vi "Counter - Read Pulse Duty Cycle and Frequency (Continuous).vi"() -> ()   [LabVIEW 2022 SP3]
doc: "This example demonstrates how to configure a Pulse measurement to acquire frequency and duty cycle based off of an external clock. \n\nThe pulse measurement feature was introduced with NI X Series and 2nd generation NI CompactDAQ devices.\n\nFor instructions on how to connect your signals to the DAQ device, refer to your device documentation."
uses:
  <vilib>/Utility/error.llb/DialogType.ctl
  <vilib>/DAQmx/read.llb/DAQmx Read (Counter 1D Pulse Freq 1 Chan NSamp).vi
  <vilib>/DAQmx/create/channels.llb/DAQmx Create Channel (CI-Pulse Freq).vi
  <vilib>/DAQmx/configure/timing.llb/DAQmx Timing (Sample Clock).vi
  <vilib>/DAQmx/miscellaneous.llb/DAQmx Fill In Error Info.vi
  <resource>/objmgr/daqmx.rc
panel:
  out "Data Array":cluster{"Duty Cycle":dbl, "Frequency":dbl}[](array[cluster])
  in  "Sample Rate":dbl=1000.0
  in  "External Clock Source":tag="PFI0"
  in  "Min Frequency":dbl=2.0 format="%0.6f"
  in  "Max Frequency":dbl=100.0 format="%0.6f"
  in  "Pulse Frequency Terminal":tag="PFI9"
  in  "Stop":bool
  in  "Samples per Loop":i32=1000
  in  "Counter":tag="Dev1/ctr0"
  # "Channel Settings"
  # "Acquired Data"
  # "Timing Settings"
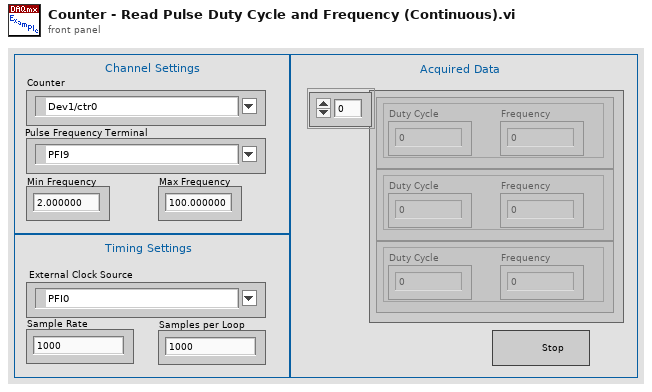
[diagram p1: front panel]
types:
  T1 = typedef "DialogType.ctl" = u16
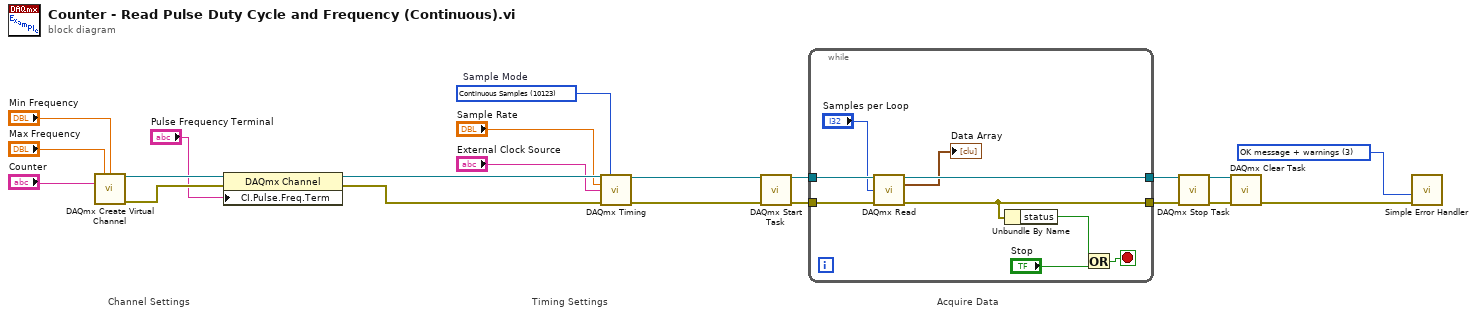
[diagram p0: block diagram]
diagram:
  w1 = T1 3 items=["no dialog", "OK message", "continue or stop message", "OK message + warnings", "continue/stop + warnings"] ("type of dialog (OK msg:1)")
  w21 = 10123 items=["Finite Samples"=10178, "Continuous Samples"=10123, "Hardware Timed Single Point"=12522]  # Sample Mode
  # "Acquire Data"
  # "Timing Settings"
  # "Channel Settings"
  n1 = call-poly <vilib>:"DAQmx Create Virtual Channel.vi"("maximum value"="Max Frequency", "minimum value"="Min Frequency", "counter"="Counter") -> ("task out"=w12:refnum<k21>, "error out"=w11:errorcluster)  [unwired: 11 in]
  n2 = property class="DAQmx Channel"(reference=w12, error in=w11, "CI.Pulse.Freq.Term"="Pulse Frequency Terminal") -> (reference out=w19:refnum<k21>, error out=w20:errorcluster)
  n3 = call-poly <vilib>:"DAQmx Timing.vi"("task/channels in"=w19, "sample mode"=w21, "rate"="Sample Rate", "source"="External Clock Source", "error in"=w20) -> ("task out"=w14:refnum<k21>, "error out"=w13:errorcluster)  [unwired: 9 in]
  n4 = call <vilib>:"DAQmx Start Task.vi"("task/channels in"=w14, "error in"=w13) -> ("task out"=w18:refnum<k21>, "error out"=w17:errorcluster)  [unwired: 12 in]
  n5 = while {
    tunnel: w18 -> [w30]
    tunnel: w17 -> [w29]
    tunnel: [w26] -> w2
    tunnel: [w27] -> w3
    stop <- w28 stop-if-true
    n6 = call-poly <vilib>:"DAQmx Read.vi"("task/channels in"=w30, "number of samples per channel"="Samples per Loop", "error in"=w29) -> ("task out"=w27:refnum<k21>, "data"=→"Data Array":cluster{"duty cycle":dbl, "frequency":dbl}[], "error out"=w26:errorcluster)  [unwired: 10 in]
    n7 = Unbundle By Name(w26) -> ("status"=w25:bool)
    n8 = Or(x=w25, y="Stop") -> (x .or. y?=w28:bool)
  }
  n9 = call <vilib>:"DAQmx Stop Task.vi"("task/channels in"=w3, "error in"=w2) -> ("task out"=w5:refnum<k21>, "error out"=w4:errorcluster)  [unwired: 12 in]
  n10 = call <vilib>:"DAQmx Clear Task.vi"("task in"=w5, "error in"=w4) -> ("error out"=w16:errorcluster)  [unwired: 13 in]
  n11 = call <vilib>:"Simple Error Handler.vi"("type of dialog (OK msg:1)"=w1, "error in (no error)"=w16) -> ()  [unwired: 3 in, 5 out]
